vi "Get Connections.vi"(8 "error in (no error)":errorcluster, 11 "RemoteControl.STM in":refnum<class "RemoteControl.STM.lvclass">) -> (0 "error out":errorcluster, 1 "Number":i32, 3 "RemoteControl.STM out":refnum<class "RemoteControl.STM.lvclass">)   [LabVIEW 2019, in "RemoteControl.STM.lvclass"]
uses:
  RemoteControl.STM.lvclass
  <vilib>/NI/STM/Connection Manager/TCP/TCP Connection Method.ctl
  RemoteControl.STM.lvclass/RemoteControl.STM.ctl
  <vilib>/NI/STM/NI STM.lvlib
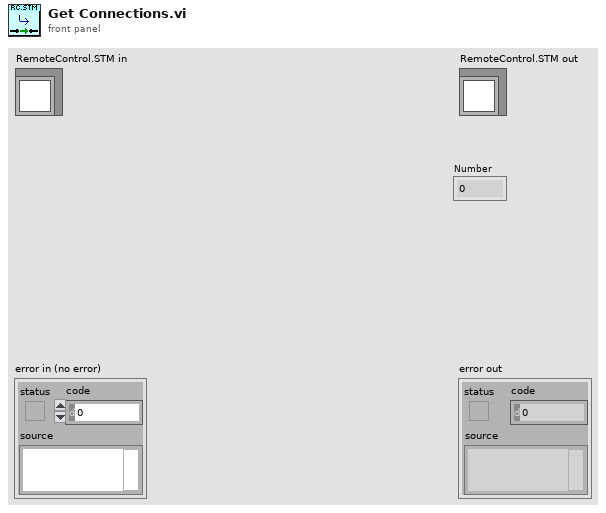
[diagram p1: front panel]
types:
  T1 = typedef "NI STM.lvlib/TCP Connection Method.ctl" = enum16{"Initialize", "Add Connection", "Set Properties", "Get Connection(s)", "Remove Connection", "Remove All Connections", "Get Connection Count"}
  T2 = typedef "NI STM.lvlib/TCP Connection Info.ctl" = cluster{"connection ID":refnum<k5>, "meta data":T3[]}
  T3 = typedef "NI STM.lvlib/MetaDataElement.ctl" = string
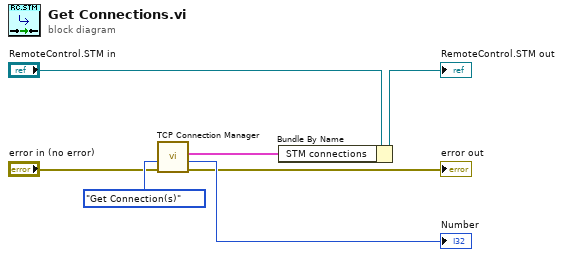
[diagram p0: block diagram]
diagram:
  n1 = call <vilib>:"TCP Connection Manager.vi"("error in"="error in (no error)", "method"=TCP_Connection_Method."Get Connection(s)") -> ("error out"=→"error out":errorcluster, "number of connections"=→"Number":i32, "all connections"=w4:T2[])  [unwired: 4 in, 3 out]
  n2 = Bundle By Name(cluster="RemoteControl.STM in", "STM connections"=w4) -> (→"RemoteControl.STM out":refnum<class "RemoteControl.STM.lvclass">)
